vi "programa 7.vi"() -> ()   [LabVIEW 2011]
panel:
  in  "Salir":bool
  in  "Suma+":bool
  out "menor":dbl
  out "mayor":dbl
  out "promedio":dbl
  out "suma":dbl
  out "Array":dbl[](array[numeric])
  in  "Generar":bool
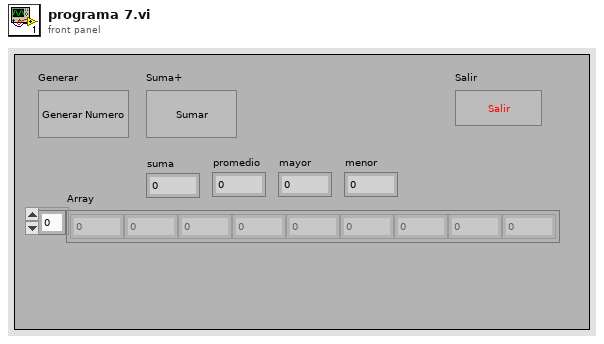
[diagram p1: front panel]
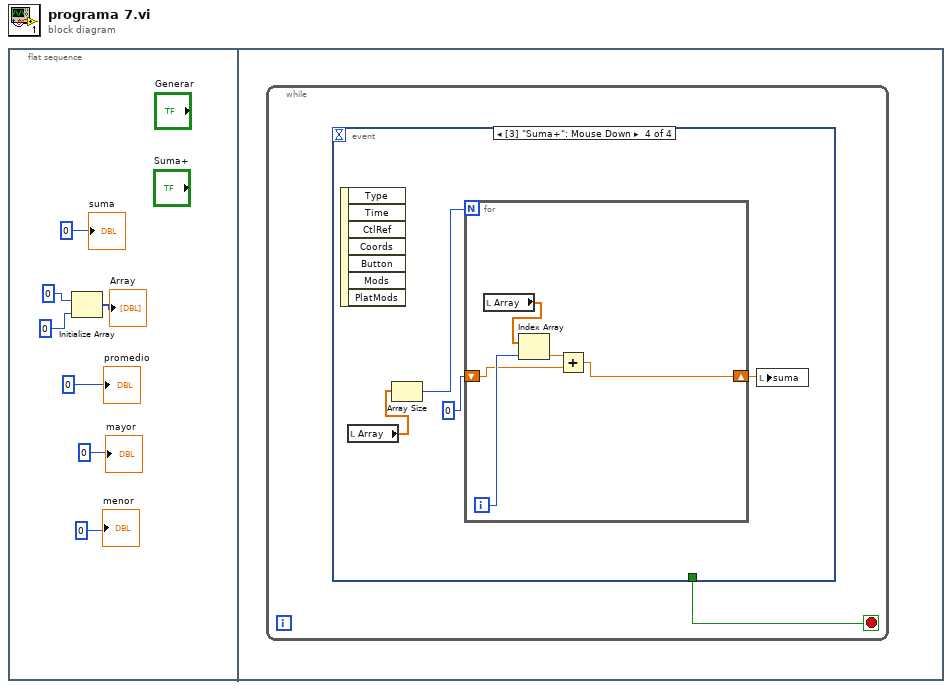
[diagram p0: block diagram]
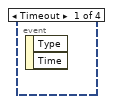
[diagram p2: hidden frame]
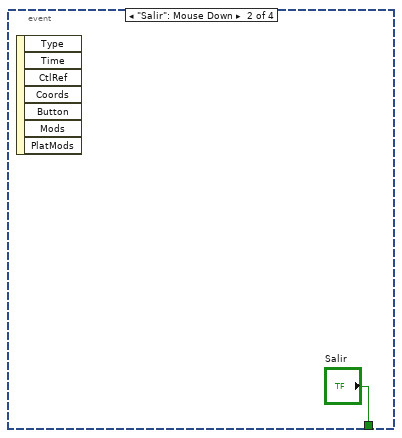
[diagram p3: hidden frame]
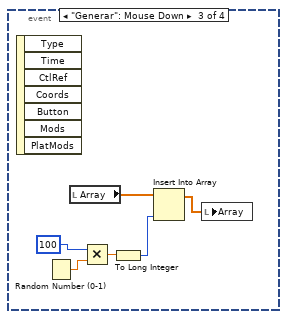
[diagram p4: hidden frame]
diagram:
  n1 = flat-sequence {
    frame #0 {
      n2 = Initialize Array(0, 0) -> (→"Array":i32[])
      "suma" <- 0
      "promedio" <- 0
      "mayor" <- 0
      "menor" <- 0
    }
    frame #1 {
      n3 = while {
        stop <- w8 stop-if-true
        n4 = event shown="[3] \"Suma+\": Mouse Down" {
          selector: _ -> [_ _ _ _]
          dyn-events: _ -> [_ _ _ _]
          timeout: _ -> [_ _ _ _]
          tunnel: [_ "Salir" _ _] -> w8
          event Timeout {
            n5 = event-data() -> ()  [unwired: 1 in, 2 out]
          }
          event "Salir": Mouse Down {
            n6 = event-data() -> ()  [unwired: 1 in, 7 out]
          }
          event "Generar": Mouse Down {
            n7 = event-data() -> ()  [unwired: 1 in, 7 out]
            n8 = Random Number (0-1)() -> (number: 0 to 1=w14:dbl)
            n9 = local read "Array"() -> (w12:dbl[])
            n10 = Multiply(x=100, y=w14) -> (x*y=w13:dbl)
            n11 = To Long Integer(number=w13) -> (32bit integer=w11:i32)
            n12 = Insert Into Array "Insert Into Array"(array=w12, new element=w11) -> (w10:dbl[])  [unwired: 1 in]
            n13 = local write "Array"(w10) -> ()
          }
          event "Suma+": Mouse Down {
            n14 = event-data() -> ()  [unwired: 1 in, 7 out]
            n15 = local read "Array"() -> (w19:dbl[])
            n16 = Array Size(array=w19) -> (size(s)=w17:i32)
            n17 = for {
              N: w17 -> [_]
              shift-right: [w20] -> w18
              shift-left: 0 -> [w21]
              i -> [w24]
              n18 = local read "Array"() -> (w23:dbl[])
              n19 = Index Array(array=w23, index=w24) -> (element=w22:dbl)
              n20 = Add(x=w22, y=w21) -> (x+y=w20:dbl)
            }
            n21 = local write "suma"(w18) -> ()
          }
        }
      }
    }
  }
